vi "Diag_8F.vi"(0 "GEA2 Reference In":refnum<k24>, 1 "Check Version?":bool, 2 "Expected Major":u8=3, 3 "Expected Minor":u8, 5 "GEA Inputs":T1 {"Destination" format="%.0x"; "Source" format="%.0x"}, 11 "Error In":errorcluster) -> (4 "GEA2 Reference Out":refnum<k24>, 6 "Major Version":u8, 8 "Minor Version":u8, 15 "Error Out":errorcluster)   [LabVIEW 2023]
uses:
  D:/Common/LabVIEW GEA2 Toolkit/source/GEA3 DLL Source/GeaCommunication.dll
  LabVIEW GEA2 Toolkit/source/GEA3 DLL Source/GeaCommunication.dll
  LabVIEW GEA2 Toolkit/GEA3/type defs/Source_Destination.ctl
  LabVIEW GEA2 Toolkit/GEA3/type defs/ERD Read Data In.ctl
  LabVIEW GEA2 Toolkit/GEA3/library/GEA2_Toolkit.lvlib
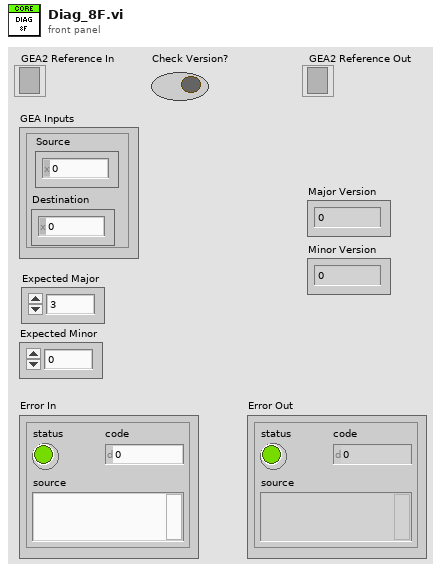
[diagram p1: front panel]
types:
  T1 = typedef "Source_Destination.ctl" = cluster{"Source":u8, "Destination":u8}
  T2 = typedef "ERD Read Data In.ctl" = cluster{"ERD Number":u16, "Data Type":enum16{"string", "boolean", "uint8_t", "uint16_t", "uint32_t", "uint64_t", "int8_t", "int16_t", "int32_t", "int64_t"}}
  T3 = typedef "ERD Read Data Out.ctl" = cluster{"ERD Number":u16, "Data":string}
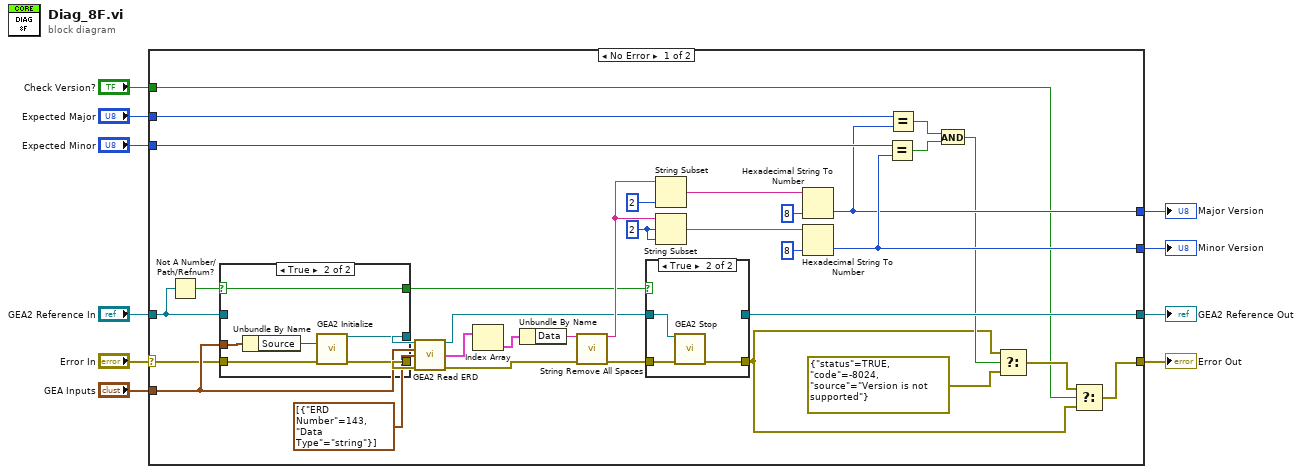
[diagram p0: block diagram]
diagram:
  n1 = case shown="No Error" "Error In" {
    selector: "Error In" -> [w18 w60]
    tunnel: "Expected Minor" -> [w44 _]
    tunnel: [w43 _] -> w9
    tunnel: "Expected Major" -> [w42 _]
    tunnel: [w41 _] -> w7
    tunnel: [w13 w60] -> w6
    tunnel: "GEA2 Reference In" -> [w40 w59]
    tunnel: "GEA Inputs" -> [w23 _]
    tunnel: "Check Version?" -> [w15 _]
    tunnel: [w19 w59] -> w2
    frame No Error {
      w39 = 2 ("offset (0)")
      n2 = Not A Number/Path/Refnum?(number/path/refnum=w40) -> (NaN/Path/Refnum?=w12:bool)
      n3 = case shown="True" w12 {
        selector: w12 -> [w50 w53]
        tunnel: w18 -> [w51 w58]
        tunnel: w23 -> [_ w57]
        tunnel: [w51 w56] -> w28
        tunnel: [w52 w55] -> w27
        tunnel: w40 -> [w52 _]
        tunnel: [w50 w53] -> w11
        frame False {
        }
        frame True {
          n4 = Unbundle By Name(w57) -> ("Source"=w54:u8)
          n5 = call "GEA2 Initialize.vi"("Source Address"=w54, "error in"=w58) -> ("GEA2 Reference Out"=w55:refnum<k24>, "error out"=w56:errorcluster)  [unwired: 10 in, 2 out]
        }
      }
      n6 = call "GEA2 Read ERD.vi"("GEA2 Reference In"=w27, "GEA Inputs"=w23, "Read ERD List"=T2[] [{"ERD Number"=143, "Data Type"=enum."string"}], "Error In"=w28) -> ("GEA2 Reference Out"=w20:refnum<k24>, "ERD Data Out"=w25:T3[], "Error Out"=w26:errorcluster)  [unwired: 8 in, 1 out]
      n7 = Index Array(array=w25) -> (element=w24:T3)  [unwired: 1 in]
      n8 = Unbundle By Name(w24) -> ("Data"=w37:string)
      n9 = call "String Remove All Spaces.vi"("Input String"=w37, "error in (no error)"=w26) -> ("Spaces Removed"=w38:string, "error out"=w21:errorcluster)  [unwired: 12 in]
      n10 = case shown="True" w11 {
        tunnel: w21 -> [w45 w49]
        tunnel: [w45 w48] -> w14
        tunnel: [w46 _] -> w19
        tunnel: w20 -> [w46 w47]
        frame False {
        }
        frame True {
          n11 = call "GEA2 Stop.vi"("GEA2 Reference In"=w47, "Error In"=w49) -> ("Error Out"=w48:errorcluster)  [unwired: 13 in]
        }
      }
      n12 = String Subset(string=w38, length (rest)=2 ("length (rest)")) -> (substring=w32:string)  [unwired: 1 in]
      n13 = String Subset(string=w38, offset (0)=w39, length (rest)=w39) -> (substring=w34:string)
      n14 = Hexadecimal String To Number(string=w32, default (0uL)=u8 8 ("default (0 U32)")) -> (number=w41:u8)  [unwired: 1 in, 1 out]
      n15 = Hexadecimal String To Number(string=w34, default (0uL)=u8 8 ("default (0 U32)")) -> (number=w43:u8)  [unwired: 1 in, 1 out]
      n16 = Equal?(x=w44, y=w43) -> (x = y?=w35:bool)
      n17 = Equal?(x=w42, y=w41) -> (x = y?=w36:bool)
      n18 = And(x=w36, y=w35) -> (x .and. y?=w16:bool)
      n19 = Select(t=w14, s=w16, f=errorcluster {"status"=TRUE, "code"=-8024, "source"="Version is not supported"} ("Error Out")) -> (s? t:f=w17:errorcluster)
      n20 = Select(t=w17, s=w15, f=w14) -> (s? t:f=w13:errorcluster)
    }
    frame Error {
    }
  }
  "Major Version" <- w7
  "Minor Version" <- w9
  "Error Out" <- w6
  "GEA2 Reference Out" <- w2
